vi "Verify Combinations.vi"(5 "Label":string, 7 "Options":refnum<class "Options.lvclass">, 8 "error in":errorcluster, 9 "ctl label -> value var[]":map{string, variant[]}(c390), 10 "VI in":refnum<vi>, 11 "LUnit Test Case In":refnum<class "Test Case.lvclass">) -> (0 "error out":errorcluster, 3 "LUnit Test Case Out":refnum<class "Test Case.lvclass">)   [LabVIEW 2020, in "LUnit.Extension.lvlib"]
doc: "This is similar to the verify parameterized (in fact it calls it behind the scenes). Instead of specifying each set of parameters, you specify a single map which maps each control label to an array of variant values (there is a utility vi, \"array to array of variants.vim) to assist with this. From this, the verify function calculates each set of parameters from all the possible combinations and verifyies each combination."
uses:
  LUnit.Extension.lvlib
  <vilib>/Astemes/LUnit/Test Case.lvclass
  Approval Tests/Options/Options.lvclass
  Approval Tests/Options/Options.lvclass/Options.ctl
  Approval Tests/Naming Data/Naming Data.lvclass/Naming Data.ctl
  <vilib>/Astemes/LUnit/Test Case.lvclass/Test Case.ctl
  Approval Tests/Approval Tests.lvlib
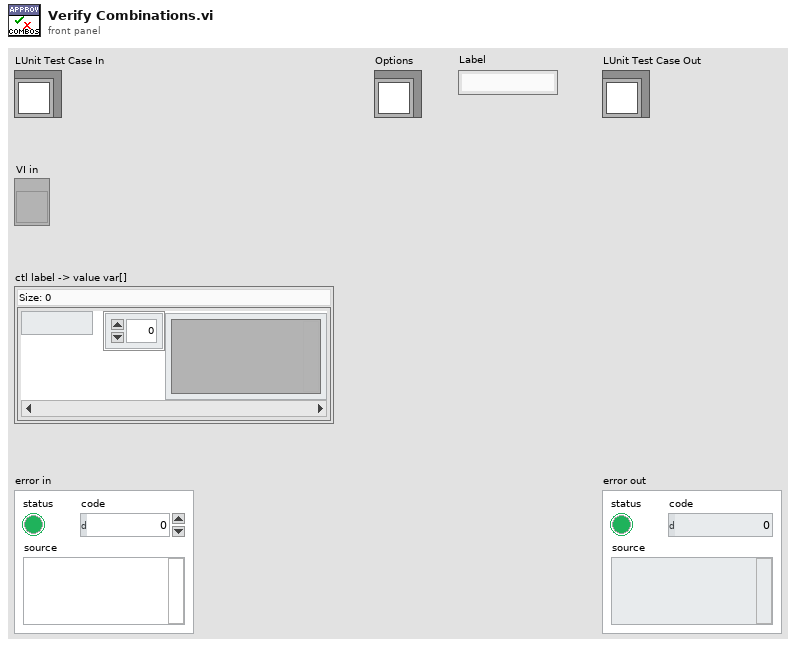
[diagram p1: front panel]
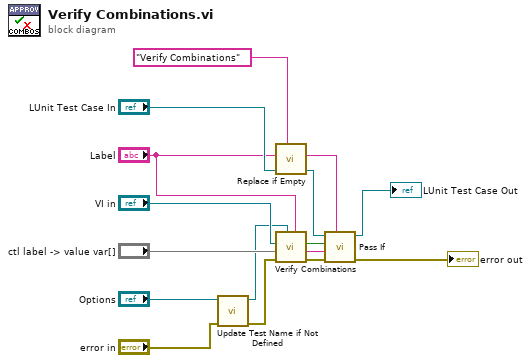
[diagram p0: block diagram]
diagram:
  n1 = call "Update Test Name if Not Defined.vi"("error in"="error in", "Options in"="Options") -> ("error out"=w12:errorcluster, "Options out"=w4:refnum<class "Options.lvclass">)  [unwired: 8 in]
  n2 = call "Replace if Empty.vi"("if empty"="Verify Combinations", "Text in"="Label") -> ("Text out"=w1:string)  [unwired: 9 in]
  n3 = call "Verify Combinations.vi"("Label"="Label", "Approval Tests.lvlib:Options.lvclass"=w4, "error in"=w12, "ctl label -> value var[]"="ctl label -> value var[]", "VI Refnum"="VI in") -> ("error out"=w13:errorcluster, "Failure Message"=w8:string, "Passed?"=w9:bool)  [unwired: 4 in]
  n4 = call <vilib>:"Pass If.vi"("Description"=w1, "error in (no error)"=w13, "Message"=w8, "Pass?"=w9, "LUnit Test Case In"="LUnit Test Case In") -> ("error out"=→"error out":errorcluster, "LUnit Test Case Out"=→"LUnit Test Case Out":refnum<class "Test Case.lvclass">)  [unwired: 5 in]
